vi "GetData.vi"(8 "error in (no error)":errorcluster, 11 "USB-9234 in":refnum<class "USB-9234.lvclass">) -> (0 "error out":errorcluster, 2 "Waveform":waveform(dbl), 3 "USB-9234 out":refnum<class "USB-9234.lvclass">)   [LabVIEW 2013, in "USB-9234.lvclass"]
uses:
  USB-9234.lvclass
  DAQSuper/DAQSuper.lvclass
  <vilib>/measure/NI_MABase.lvlib
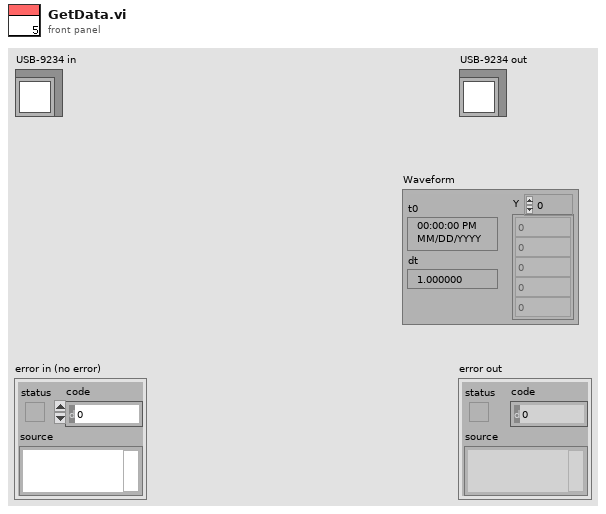
[diagram p1: front panel]
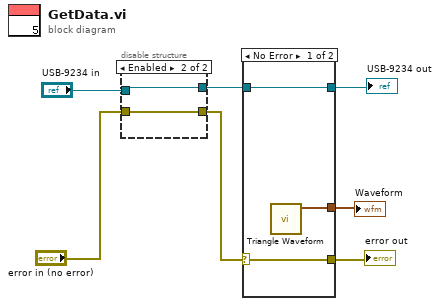
[diagram p0: block diagram]
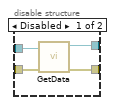
[diagram p3: hidden frame]
diagram:
  n1 = disable-structure shown="Enabled" {
    disable-tunnel: [w11 w12] -> w5
    disable-tunnel: [w10 w13] -> w3
    disable-tunnel: "error in (no error)" -> [w9 w12]
    disable-tunnel: "USB-9234 in" -> [w8 w13]
    frame Disabled {
      n2 = call-parent "GetData.vi"("error in (no error)"=w9, "DAQSuper in"=w8) -> ("error out"=w11:errorcluster, "DAQSuper out"=w10:refnum<class "USB-9234.lvclass">)  [unwired: 7 in, 1 out]
    }
    frame Enabled {
    }
  }
  n3 = case shown="No Error" w5 {
    selector: w5 -> [w16 w17]
    tunnel: [w16 w17] -> w4
    tunnel: w3 -> [w15 w18]
    tunnel: [w15 w18] -> w2
    tunnel: [w14 _] -> w1
    frame No Error {
      n4 = call <vilib>:"Triangle Waveform.vi"() -> ("signal out"=w14:waveform(dbl))  [unwired: 10 in, 1 out]
    }
    frame Error {
    }
  }
  "error out" <- w4
  "USB-9234 out" <- w2
  "Waveform" <- w1
